vi "Keithley 6514 Set & Enable SRQ.vi"(0 "Resource In":refnum<visa-resource-name>, 1 "Check For SCPI Errors? (T)":bool=TRUE, 5 "OSB":bool, 7 "ESB":bool, 9 "MAV":bool, 11 "error in (no error)":T1, 12 "QSB":bool, 13 "EAV":bool, 14 "MSB":bool) -> (4 "Resource Out (dupl)":refnum<visa-resource-name>, 15 "error out":T1)   [LabVIEW 2014, in "KE6514Driver.lvlib"]
doc: "This VI is used to enable the various bits for SRQing the Instrument\n\nMSB = Measurement Summary Bit\nTrue = On with value of 1\nFalse = Off with value of 0\n\nEAV = Error Available Bit\nTrue = On with value of 4\nFalse = Off with value of 0\n\nQSB = Questionable Summary Bit\nTrue = On with value of 8\nFalse = Off with value of 0\n\nMAV = Message Available Bit\nTrue = On with value of 16\nFalse = Off with value of 0\n\nESB = Event Summary Bit\nTrue = On with value of 32\nFalse = Off with value of 0\n\nOSB = Operation Summary Bit\nTrue = On with value of 128\nFalse = Off with value of 0"
uses:
  KE6514Driver.lvlib
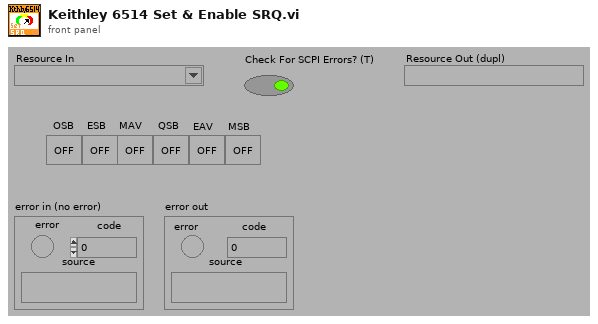
[diagram p1: front panel]
types:
  T1 = cluster{"error":bool, "code":i32, "source":string}
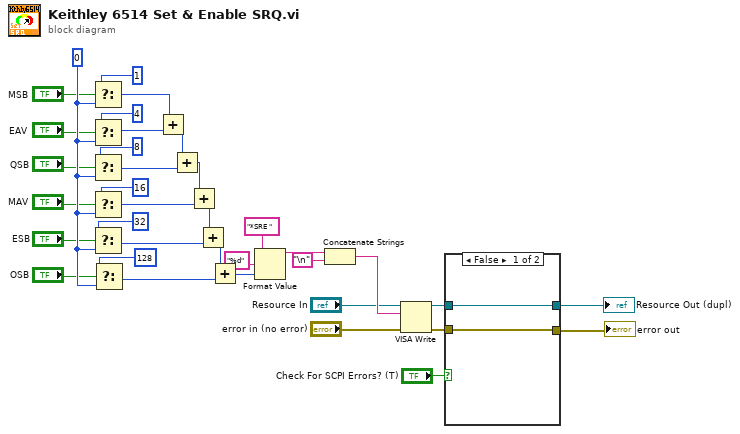
[diagram p0: block diagram]
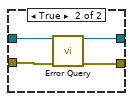
[diagram p2: hidden frame]
diagram:
  w22 = 0
  n1 = Select(t=1, s="MSB", f=w22) -> (s? t:f=w31:i32)
  n2 = Select(t=4, s="EAV", f=w22) -> (s? t:f=w30:i32)
  n3 = Select(t=8, s="QSB", f=w22) -> (s? t:f=w33:i32)
  n4 = Select(t=16, s="MAV", f=w22) -> (s? t:f=w35:i32)
  n5 = Select(t=32, s="ESB", f=w22) -> (s? t:f=w28:i32)
  n6 = Select(t=128, s="OSB", f=w22) -> (s? t:f=w23:i32)
  n7 = Add(x=w31, y=w30) -> (x+y=w32:i32)
  n8 = Add(x=w32, y=w33) -> (x+y=w34:i32)
  n9 = Add(x=w34, y=w35) -> (x+y=w36:i32)
  n10 = Add(x=w36, y=w28) -> (x+y=w20:i32)
  n11 = Add(x=w20, y=w23) -> (x+y=w13:i32)
  n12 = Format Value(string ("")="*SRE ", format string="%d", value (0)=w13) -> (output string=w10:string)
  n13 = Concatenate Strings(w10, "\n") -> (w8:string)
  n14 = VISA Write(VISA resource name="Resource In", write buffer=w8, error in (no error)="error in (no error)") -> (VISA resource name out=w4:refnum<visa-resource-name>, error out=w3:errorcluster)  [unwired: 1 out]
  n15 = case shown="False" "Check For SCPI Errors? (T)" {
    tunnel: w4 -> [w38 w42]
    tunnel: w3 -> [w37 w41]
    tunnel: [w37 w40] -> w1
    tunnel: [w38 w39] -> w2
    frame False {
    }
    frame True {
      n16 = call "Error Query.vi"("VISA Resource In"=w42, "error in (no error)"=w41) -> ("VISA Resource Out (dupl)"=w39:refnum<visa-resource-name>, "error out"=w40:errorcluster)  [unwired: 10 in, 2 out]
    }
  }
  "error out" <- w1
  "Resource Out (dupl)" <- w2
